vi "Write Key.vi"(8 "error in":errorcluster, 9 "value":string, 10 "key":string, 11 "Configuration in":refnum<class "Configuration.lvclass">) -> (0 "error out":errorcluster, 3 "Configuration out":refnum<class "Configuration.lvclass">)   [LabVIEW 2018, in "Configuration.lvlib" / "Configuration.lvclass"]
doc: "Used to update the key values in a config.ini file."
uses:
  Configuration.lvclass
  Configuration.lvclass/Configuration.ctl
  <vilib>/Utility/config.llb/Write Key (String).vi
  <vilib>/Utility/config.llb/NI_LVConfig.lvlib
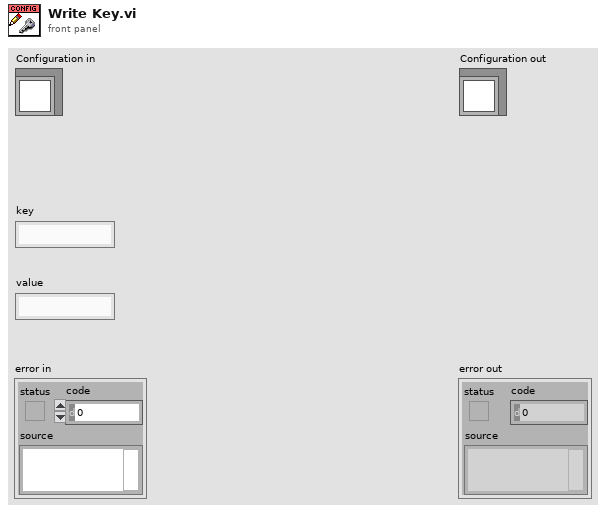
[diagram p1: front panel]
types:
  T1 = typedef "NI_LVConfig.lvlib/Config Data RefNum.ctl" = refnum<k1>
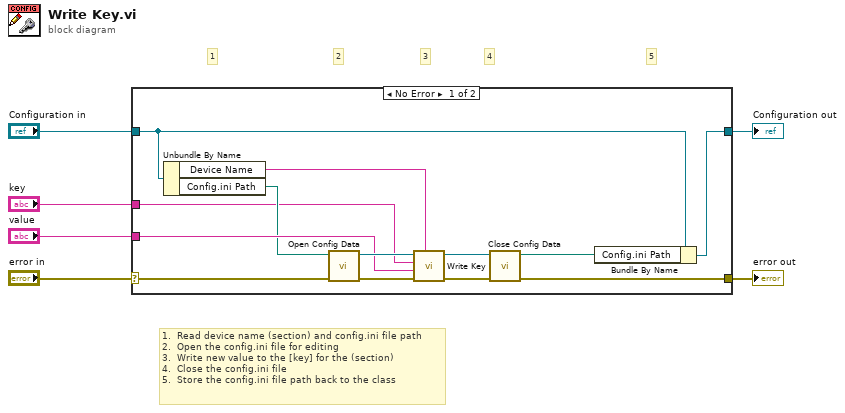
[diagram p0: block diagram]
diagram:
  # "1.  Read device name (section) and config.ini file path\n2.  Open the config.ini file for editing\n3.  Write new value to the [key] for the (section)\n4.  Close the config.ini file\n5.  Store the config.ini file path back to the class"
  # "5"
  # "4"
  # "3"
  # "2"
  # "1"
  n1 = case shown="No Error" "error in" {
    selector: "error in" -> [w12 w21]
    tunnel: [w11 w21] -> w5
    tunnel: [w10 w20] -> w3
    tunnel: "Configuration in" -> [w14 w20]
    tunnel: "key" -> [w7 _]
    tunnel: "value" -> [w15 _]
    frame No Error {
      n2 = Unbundle By Name(w14) -> ("Device Name"=w8:string, "Config.ini Path"=w13:path)
      n3 = call <vilib>:"Open Config Data.vi"("error in (no error)"=w12, "configuration file path"=w13) -> ("error out"=w18:errorcluster, "refnum"=w19:T1)  [unwired: 7 in, 1 out]
      n4 = call-poly <vilib>:"Write Key.vi"("section"=w8, "error in (no error)"=w18, "value"=w15, "key"=w7, "refnum"=w19) -> ("error out"=w17:errorcluster, "refnum out"=w16:T1)  [unwired: 4 in, 1 out]
      n5 = call <vilib>:"Close Config Data.vi"("error in (no error)"=w17, "refnum"=w16) -> ("error out"=w11:errorcluster, "file path"=w9:path)  [unwired: 8 in]
      n6 = Bundle By Name(cluster=w14, "Config.ini Path"=w9) -> (w10:refnum<class "Configuration.lvclass">)
    }
    frame Error {
    }
  }
  "error out" <- w5
  "Configuration out" <- w3
